vi "Drive Set.vi"(1 "Set In":T1) -> ()   [LabVIEW 2016]
uses:
  <vilib>/Rock Robotics/WPI/Utilities/WPI_GetSetVariantRefNum.vi
  <vilib>/Rock Robotics/WPI/Solenoid/Deprecated/WPI_SolenoidSetBool.vi
panel:
  out "Set Out":T1
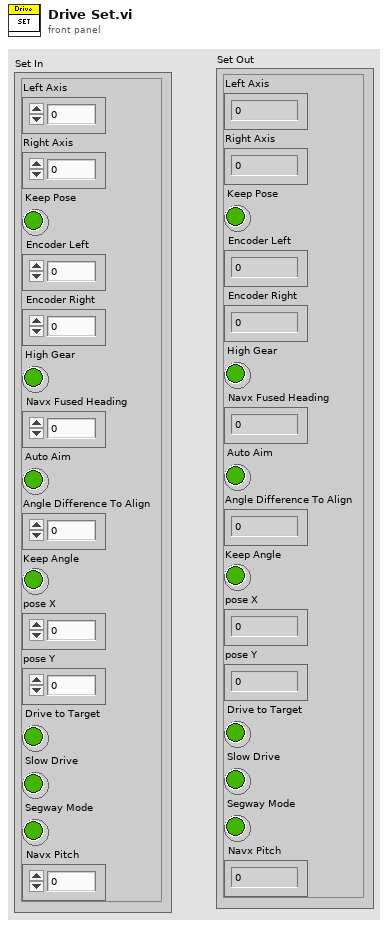
[diagram p1: front panel]
types:
  T1 = cluster{"Left Axis":dbl, "Right Axis":dbl, "Keep Pose":bool, " Encoder Left":dbl, " Encoder Right":dbl, "High Gear":bool, " Navx Fused Heading":dbl, "Auto Aim":bool, "Angle Difference To Align":dbl, "Keep Angle":bool, "pose X":dbl, "pose Y":dbl, "Drive to Target":bool, "Slow Drive":bool, "Segway Mode":bool, " Navx Pitch":dbl}
  T2 = typedef "WPI_SolenoidDevRef.ctl" = cluster{"DevStatus":errorcluster, "Pneumatics Control Module":u8, "Forward Solenoid Channel":T3, "Reverse Solenoid Channel":T3}
  T3 = typedef "WPI_SolenoidChannel.ctl" = enum8{"Solenoid 0", "Solenoid 1", "Solenoid 2", "Solenoid 3", "Solenoid 4", "Solenoid 5", "Solenoid 6", "Solenoid 7", "Invalid"}
  T4 = typedef "WPI_RobotDriveDevRef.ctl" = cluster{"DevStatus":errorcluster, "Motors[]":T5[], "Square Inputs":bool, "Max Output":dbl}
  T5 = typedef "WPI_MotorControlDeviceRef.ctl" = cluster{"DeviceStatus":errorcluster, "Type":T6, "PWM":cluster{"PWM Channel":T7, "DeadBand":T8}, "CAN":cluster{"Device Number":u8, "SetOutput VI Ref":variant, "GetOutput VI Ref":variant, "Enable VI Ref":variant, "Disable VI Ref":variant, "Data":variant}, "Invert":bool}
  T6 = typedef "WPI_MotorControlType.ctl" = enum16{"PWM", "CAN"}
  T7 = typedef "FPGA_DIOPWMChannel.ctl" = enum8{"PWM 0", "PWM 1", "PWM 2", "PWM 3", "PWM 4", "PWM 5", "PWM 6", "PWM 7", "PWM 8", "PWM 9", "PWM MXP 0", "PWM MXP 1", "PWM MXP 2", "PWM MXP 3", "PWM MXP 4", "PWM MXP 5", "PWM MXP 6", "PWM MXP 7", "PWM MXP 8", "PWM MXP 9", "Invalid"}
  T8 = typedef "WPI_PWMDeadband.ctl" = cluster{"Name":string, "maxPositivePwm":i32, "minPositivePwm":i32, "centerPwm":i32, "maxNegativePwm":i32, "minNegativePwm":i32, "angularRange":u16}
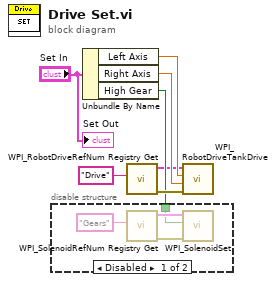
[diagram p0: block diagram]
diagram:
  n1 = Unbundle By Name("Set In") -> ("Left Axis"=w4:dbl, "Right Axis"=w3:dbl, "High Gear"=w5:bool)
  n2 = disable-structure shown="Disabled" {
    disable-tunnel: w5 -> [w8 _]
    frame Disabled {
      n3 = call <vilib>:"WPI_SolenoidRefNum Registry Get.vi"("refnum name"="Gears") -> ("error out"=w11:errorcluster, "SolenoidDevRef"=w10:T2)  [unwired: 9 in]
      n4 = call-poly <vilib>:"WPI_SolenoidSet.vi"("error in (no error)"=w11, "Value"=w8, "SolenoidDevRef"=w10) -> ()  [unwired: 7 in, 2 out]
    }
    frame Enabled {
    }
  }
  n5 = call <vilib>:"WPI_RobotDriveRefNum Registry Get.vi"("refnum name"="Drive") -> ("error out"=w7:errorcluster, "RobotDriveDevRef"=w2:T4)  [unwired: 9 in]
  n6 = call <vilib>:"WPI_RobotDriveTankDrive.vi"("error in (no error)"=w7, "Right axis value"=w3, "Left axis value"=w4, "RobotDriveDevRef"=w2) -> ()  [unwired: 5 in, 3 out]
  "Set Out" <- "Set In"
